vi "Create Channel Arrays.vi"(0 "Display State In":T2={"Current Channels Info"=[], "Help Prefix"="", "Max Display Size"=8, "Max Size"=0, "Show Buttons"=TRUE, "Data Valid"=refnum, "Show Range"=FALSE, "Range Items"=[], "Range Index"=[]}, 9 "Container State":T5, 11 "error in (no error)":errorcluster) -> (3 "Range Indexes":i32[](array[numeric]), 4 "Display State Out":T2={"Current Channels Info"=[], "Help Prefix"="", "Max Display Size"=8, "Max Size"=0, "Show Buttons"=TRUE, "Data Valid"=refnum, "Show Range"=FALSE, "Range Items"=[], "Range Index"=[]}, 6 "Channel Names":string[](array[string]), 8 "Channel Aliases":string[](array[string]), 10 "Connection Informations":T1(array[cluster]), 15 "error out":errorcluster)   [LabVIEW 2021, in "myRIO Channel List.xctl"]
uses:
  <vilib>/myRIO/Common/Express VI Framework/xctls/myRIO Channel List/myRIO Channel List.xctl
  <vilib>/_xctls/Container State.ctl
  <vilib>/myRIO/Common/Express VI Framework/xctls/myRIO Channel List/State.ctl
  <vilib>/myRIO/Common/Profile Manager Framework/typedefs/Channel Info.ctl
  <vilib>/myRIO/Common/Express VI Framework/typedefs/Data Validate Ref.ctl
  <vilib>/myRIO/Common/Express VI Framework/xctls/myRIO Channel List/typedefs/Channel Typedef.ctl
  <vilib>/_xctls/XControlSupport.lvlib
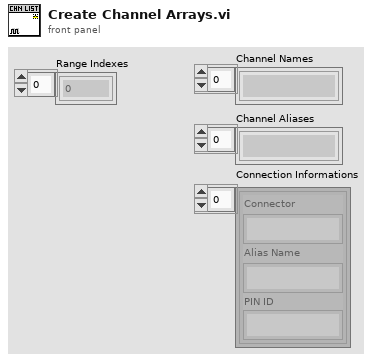
[diagram p1: front panel]
types:
  T1 = cluster{"Connector":string, "Alias Name":string, "PIN ID":string}[]
  T2 = typedef "myRIO Channel List.xctl/State.ctl" = cluster{"Current Channels Info":T3[], "Help Prefix":string, "Max Display Size":i32, "Max Size":i32, "Show Buttons":bool, "Data Valid":T4, "Show Range":bool, "Range Items":string[], "Range Index":i32[]}
  T3 = typedef "Channel Info.ctl" = cluster{"Channel Name":string, "Alias":string, "Used?":bool, "Not Support?":bool, "Property Bundle":cluster{"Name":string, "Value":variant}[]}
  T4 = typedef "Data Validate Ref.ctl" = refnum<user-event>
  T5 = typedef "XControlSupport.lvlib/Container State.ctl" = cluster{"Indicator?":bool, "Run Mode?":bool, " Refnum":refnum<vi>}
  T6 = cluster{"Connector":string, "Alias Name":string, "PIN ID":string}
  T7 = typedef "Channel Typedef.ctl" = cluster{"Channel Name":u16, "Channel Alias":string, "Delete Channel":bool, "Index":i32}
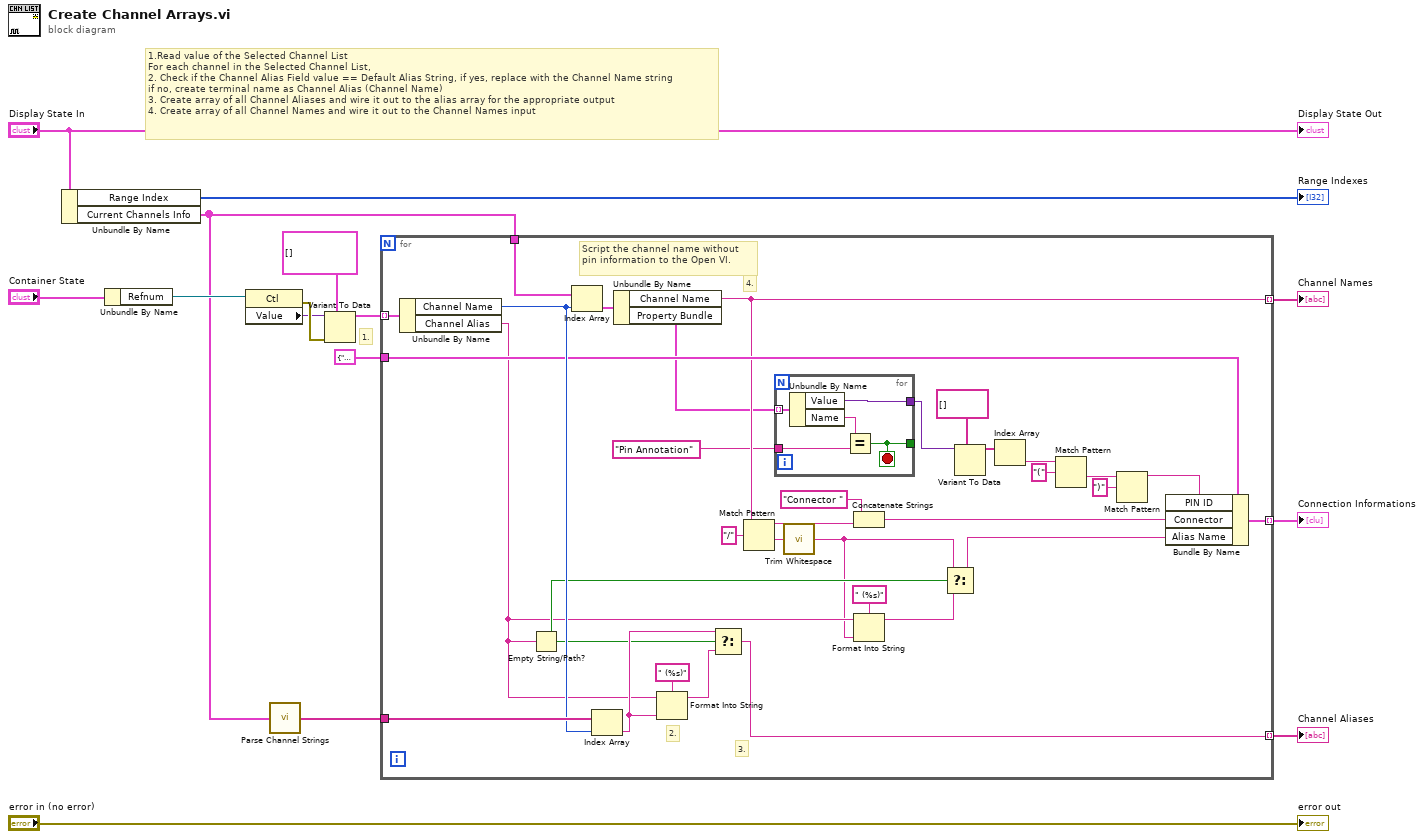
[diagram p0: block diagram]
diagram:
  # "1.Read value of the Selected Channel List\nFor each channel in the Selected Channel List, \n2. Check if the Channel Alias Field value == Default Alias String, if yes, replace with the Channel Name string\nif no, create terminal name as Channel Alias (Channel Name)\n3. Create array of all Channel Aliases and wire it out to the alias array for the appropriate output\n4. Create array of all Channel Names and wire it out to the Channel Names input"
  # "1."
  n1 = Unbundle By Name("Display State In") -> ("Range Index"=→"Range Indexes":i32[], "Current Channels Info"=w2:T3[])
  n2 = Unbundle By Name("Container State") -> ("Refnum"=w12:refnum<vi>)
  n3 = property class="Ctl"(reference=w12) -> (error out=w11:errorcluster, "Value"=w10:variant)  [unwired: 1 in, 1 out]
  n4 = call <vilib>:"Parse Channel Strings.vi"("Channels Info"=w2) -> ("Channel Strings"=w3:string[])
  n5 = Variant To Data(error in=w11, type=T7[] [] ("Selected"), Variant=w10) -> (data=w14:T7[])  [unwired: 1 out]
  n6 = for {
    tunnel: w14 -> [w48] mode=indexing
    tunnel: [w39] -> w7 mode=indexing
    tunnel: [w26] -> w6 mode=indexing
    tunnel: w3 -> [w46]
    tunnel: w2 -> [w42]
    tunnel: T6 {"Connector"="", "Alias Name"="", "PIN ID"=""} ("Connection Information") -> [w40]
    tunnel: [w36] -> w5 mode=indexing
    # "Script the channel name without pin information to the Open VI."
    # "3."
    # "4."
    # "2."
    n7 = Unbundle By Name(w48) -> ("Channel Name"=w45:u16, "Channel Alias"=w28:string)
    n8 = Empty String/Path?(string/path=w28) -> (empty?=w33:bool)
    n9 = Index Array(array=w42, index=w45) -> (element=w41:T3)
    n10 = Index Array(array=w46, index=w45) -> (element=w43:string)
    n11 = Unbundle By Name(w41) -> ("Channel Name"=w39:string, "Property Bundle"=w18:cluster{"Name":string, "Value":variant}[])
    n12 = Format Into String(format string=" (%s)", initial string=w28, w43) -> (resulting string=w44:string)  [unwired: 1 in, 1 out]
    n13 = Select(t=w43, s=w33, f=w44) -> (s? t:f=w26:string)
    n14 = Match Pattern(string=w39, regular expression="/") -> (before substring=w37:string, after substring=w30:string)  [unwired: 1 in, 2 out]
    n15 = for {
      tunnel: w18 -> [w53] mode=indexing
      tunnel: "Pin Annotation" ("x") -> [w51]
      tunnel: [w50] -> w16
      tunnel: [w49] -> _
      stop <- w49 stop-if-true
      n16 = Unbundle By Name(w53) -> ("Value"=w50:variant, "Name"=w52:string)
      n17 = Equal?(x=w52, y=w51) -> (x = y?=w49:bool)
    }
    n18 = call <vilib>:"Trim Whitespace.vi"("string"=w30) -> ("trimmed string"=w27:string)  [unwired: 1 in]
    n19 = Concatenate Strings("Connector " ("string"), w37) -> (w32:string)
    n20 = Format Into String(format string=" (%s)", initial string=w28, w27) -> (resulting string=w34:string)  [unwired: 1 in, 1 out]
    n21 = Select(t=w27, s=w33, f=w34) -> (s? t:f=w29:string)
    n22 = Variant To Data(type=string[] [], Variant=w16) -> (data=w24:string[])  [unwired: 1 in, 1 out]
    n23 = Index Array(array=w24) -> (element=w23:string)  [unwired: 1 in]
    n24 = Match Pattern(string=w23, regular expression="(") -> (after substring=w21:string)  [unwired: 1 in, 3 out]
    n25 = Match Pattern(string=w21, regular expression=")") -> (before substring=w19:string)  [unwired: 1 in, 3 out]
    n26 = Bundle By Name(cluster=w40, "PIN ID"=w19, "Connector"=w32, "Alias Name"=w29) -> (w36:T6)
  }
  "Channel Names" <- w7
  "Channel Aliases" <- w6
  "Connection Informations" <- w5
  "Display State Out" <- "Display State In"
  "error out" <- "error in (no error)"
